vi "LVClass_ComputePhaseSet SetZonalFilter.vi"(0 "ComputePhaseSet in":refnum<class "ComputePhaseSet.lvclass">, 5 "numero_zonal_to_filter":u8[](array[numeric]), 11 "error in (no error)":errorcluster) -> (4 "ComputePhaseSet out":refnum<class "ComputePhaseSet.lvclass">, 15 "error out":errorcluster)   [LabVIEW 2020, in "ComputePhaseSet.lvclass"]
doc: "Set filter for zonal phase reconstruction. The aberrations to filter are\nselected using the boolean values in the params array. (0 = aberration is\nremoved).\n\n<B>ComputePhaseSetIn</B> : ComputePhaseSet object.\n<B>ComputePhaseSetOut</B> : ComputePhaseSet object.\n<B>params</B> : Array of aberrations to filter."
uses:
  ComputePhaseSet.lvclass
  ComputePhaseSet.lvclass/ComputePhaseSet.ctl
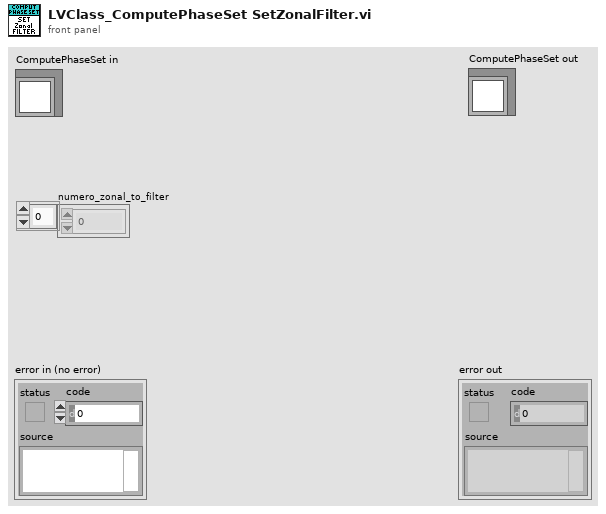
[diagram p1: front panel]
types:
  T1 = typedef "ClassID.ctl" = i64
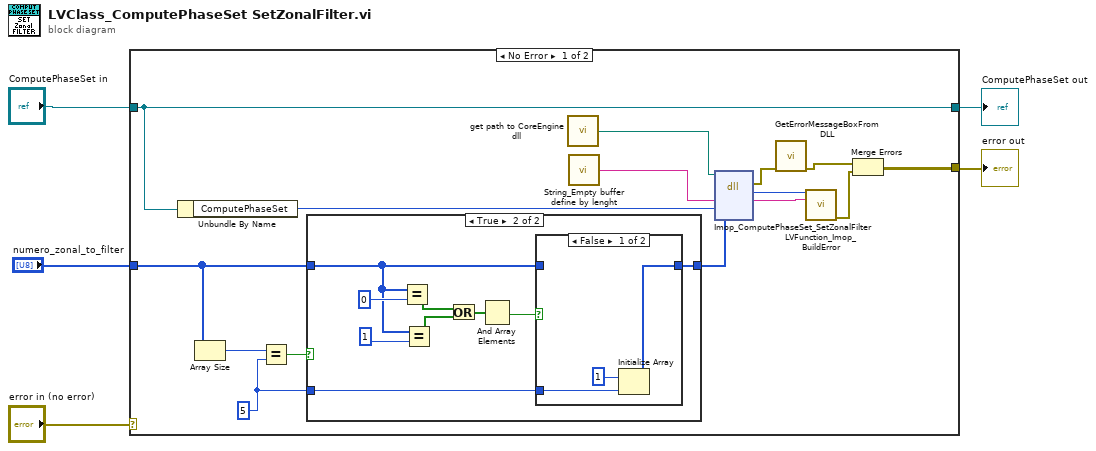
[diagram p0: block diagram]
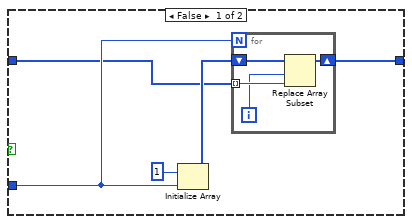
[diagram p2: hidden frame]
diagram:
  n1 = case shown="No Error" "error in (no error)" {
    selector: "error in (no error)" -> [_ w44]
    tunnel: [w6 w44] -> w2
    tunnel: [w14 w43] -> w4
    tunnel: "ComputePhaseSet in" -> [w14 w43]
    tunnel: "numero_zonal_to_filter" -> [w11 _]
    frame No Error {
      w9 = 5 ("y")
      n2 = Unbundle By Name(w14) -> ("ComputePhaseSet"=w15:T1)
      n3 = Array Size(array=w11) -> (size(s)=w13:i32)
      n4 = Equal?(x=w13, y=w9) -> (x = y?=w12:bool)
      n5 = case shown="True" w12 {
        tunnel: w11 -> [w21 w32]
        tunnel: [w23 w31] -> w10
        tunnel: w9 -> [w22 w30]
        frame False {
          n6 = Initialize Array(u8 1, w22) -> (w24:u8[])
          n7 = for {
            N: w22 -> [_]
            shift-right: [w28] -> w23
            shift-left: w24 -> [w29]
            tunnel: w21 -> [w27] mode=indexing
            i -> [w26]
            n8 = Replace Array Subset(array=w29, new element=w27, index=w26) -> (w28:u8[])
          }
        }
        frame True {
          n9 = Equal?(x=w32, y=0) -> (x = y?=w36:bool[])
          n10 = Equal?(x=w32, y=1) -> (x = y?=w35:bool[])
          n11 = Or(x=w36, y=w35) -> (x .or. y?=w34:bool[])
          n12 = And Array Elements(Boolean array=w34) -> (logical AND=w33:bool)
          n13 = case shown="False" w33 {
            tunnel: w32 -> [_ w42]
            tunnel: [w39 w42] -> w31
            tunnel: w30 -> [w40 _]
            frame False {
              n14 = Initialize Array(u8 1, w40) -> (w39:u8[])
            }
            frame True {
            }
          }
        }
      }
      n15 = call "get path to CoreEngine dll.vi"() -> ("path to wavekit library"=w17:path)  [unwired: 14 in, 1 out]
      n16 = call "String_Empty buffer define by lenght.vi"() -> ("Empty buffer"=w18:string)  [unwired: 1 in]
      n17 = dll-call lib="D:/2_trunk/Soft_haso/ImOpCoreEngine4_LV2011/DLLs/ImopEngine4_vc100.dll" fn="Imop_ComputePhaseSet_SetZonalFilter"(path in=w17, "message"=w18, "objet"=w15, "param"=w10) -> (error out=w16:errorcluster, "return type"=w20:i32, "message"=w19:string)  [unwired: 4 in, 1 out]
      n18 = call "GetErrorMessageBoxFromDLL.vi"("error IN"=w16) -> ("error OUT"=w8:errorcluster)  [unwired: 10 in]
      n19 = call "LVFunction_Imop_BuildError.vi"("code"=w20, "String to Prepend to source (\"\")"=w19) -> ("error out"=w7:errorcluster)  [unwired: 13 in]
      n20 = Merge Errors(w8, w7) -> (w6:errorcluster)
    }
    frame Error {
    }
  }
  "error out" <- w2
  "ComputePhaseSet out" <- w4
